vi "filename_stl.vi"(11 "Received":string) -> (3 "appended path":path)   [LabVIEW 2019]
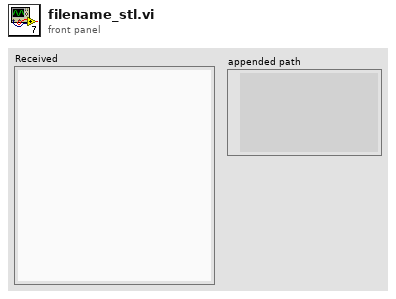
[diagram p1: front panel]
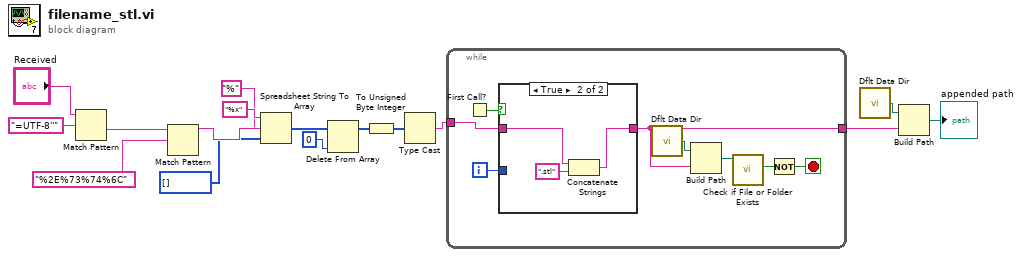
[diagram p0: block diagram]
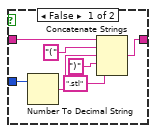
[diagram p2: hidden frame]
diagram:
  n1 = Match Pattern(string="Received", regular expression="=UTF-8''") -> (after substring=w7:string)  [unwired: 1 in, 3 out]
  n2 = Match Pattern(string=w7, regular expression="%2E%73%74%6C") -> (before substring=w13:string)  [unwired: 1 in, 3 out]
  n3 = Spreadsheet String To Array(delimiter (Tab)="%", format string="%x", spreadsheet string=w13, array type (2D Dbl)=i32[] []) -> (array=w14:i32[])
  n4 = Delete From Array(array=w14, index=0 ("length")) -> (array with subset deleted=w16:i32[])  [unwired: 1 in, 1 out]
  n5 = To Unsigned Byte Integer(number=w16) -> (unsigned 8bit integer=w12:u8[])
  n6 = Type Cast(x=w12) -> (*(type *) &x=w2:string)  [unwired: 1 in]
  n7 = while {
    tunnel: w2 -> [w18]
    tunnel: [w17] -> w1
    i -> [w19]
    stop <- w21 stop-if-true
    n8 = First Call?() -> (First Call?: T/F=w20:bool)
    n9 = case shown="True" w20 {
      tunnel: w19 -> [w31 _]
      tunnel: w18 -> [w30 w34]
      tunnel: [w29 w32] -> w17
      frame False {
        n10 = Number To Decimal String(number=w31) -> (decimal integer string=w28:string)  [unwired: 1 in]
        n11 = Concatenate Strings(w30, "(" ("string"), w28, ")" ("string"), ".stl" ("string")) -> (w29:string)
      }
      frame True {
        n12 = Concatenate Strings(w34, ".stl" ("string")) -> (w32:string)
      }
    }
    n13 = call <vilib>:"Dflt Data Dir.vi"() -> ("App:Default Data Directory"=w23:path)
    n14 = Build Path(base path=w23, name or relative path=w17) -> (appended path=w24:path)
    n15 = call <vilib>:"Check if File or Folder Exists.vi"("path"=w24) -> ("file or folder exists?"=w22:bool)  [unwired: 8 in, 2 out]
    n16 = Not(x=w22) -> (.not. x?=w21:bool)
  }
  n17 = call <vilib>:"Dflt Data Dir.vi"() -> ("App:Default Data Directory"=w4:path)
  n18 = Build Path(base path=w4, name or relative path=w1) -> (appended path=→"appended path":path)
